vi "Call_SubPanal.vi"(8 "错误输入（无错误）":errorcluster, 10 "VI引用句柄":refnum<vi>, 11 "SubPnl引用句柄":refnum<vi>) -> (0 "错误输出":errorcluster)   [LabVIEW 2020]
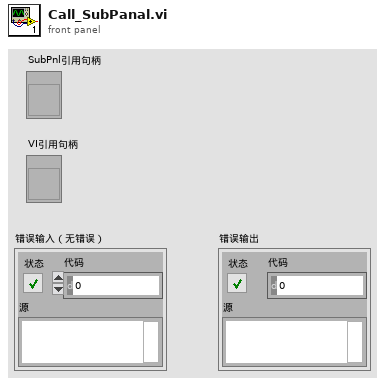
[diagram p1: front panel]
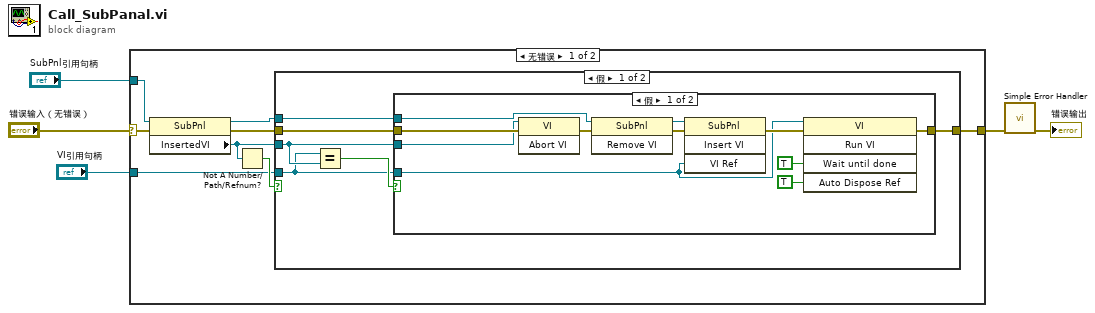
[diagram p0: block diagram]
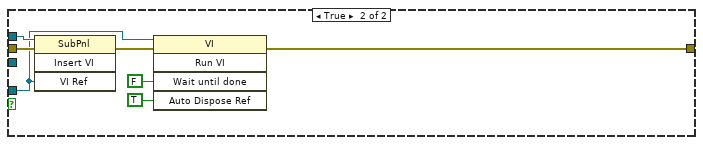
[diagram p3: hidden frame]
diagram:
  n1 = case shown="无错误" "错误输入（无错误）" {
    selector: "错误输入（无错误）" -> [w8 w39]
    tunnel: "SubPnl引用句柄" -> [w9 _]
    tunnel: "VI引用句柄" -> [w7 _]
    tunnel: [w6 w39] -> w2
    frame No Error {
      n2 = property class="SubPnl"(reference=w9, error in=w8) -> (reference out=w11:refnum<vi>, error out=w10:errorcluster, "InsertedVI"=w12:refnum<vi>)
      n3 = Not A Number/Path/Refnum?(number/path/refnum=w12) -> (NaN/Path/Refnum?=w13:bool)
      n4 = case shown="假" w13 {
        tunnel: w12 -> [w17 _]
        tunnel: w11 -> [w19 w37]
        tunnel: w10 -> [w18 w38]
        tunnel: w7 -> [w15 w35]
        tunnel: [w14 w32] -> w6
        frame False {
          n5 = Equal?(x=w15, y=w17) -> (x = y?=w16:bool)
          n6 = case shown="假" w16 {
            tunnel: w19 -> [w30 _]
            tunnel: w18 -> [w28 w31]
            tunnel: w17 -> [w27 _]
            tunnel: w15 -> [w23 _]
            tunnel: [w20 w31] -> w14
            frame False {
              n7 = invoke class="VI" method="Abort VI"(reference=w27, error in=w28) -> (error out=w29:errorcluster)  [unwired: 1 in, 2 out]
              n8 = invoke class="SubPnl" method="Remove VI"(reference=w30, error in=w29) -> (reference out=w25:refnum<vi>, error out=w26:errorcluster)  [unwired: 1 in, 1 out]
              n9 = invoke class="SubPnl" method="Insert VI"(reference=w25, error in=w26, "VI Ref"=w23) -> (error out=w24:errorcluster)  [unwired: 1 in, 3 out]
              n10 = invoke class="VI" method="Run VI"(reference=w23, error in=w24, "Wait until done"=TRUE ("结束前等待"), "Auto Dispose Ref"=TRUE ("自动销毁引用")) -> (error out=w20:errorcluster)  [unwired: 1 in, 4 out]
            }
            frame True {
            }
          }
        }
        frame True {
          n11 = invoke class="SubPnl" method="Insert VI"(reference=w37, error in=w38, "VI Ref"=w35) -> (error out=w36:errorcluster)  [unwired: 1 in, 3 out]
          n12 = invoke class="VI" method="Run VI"(reference=w35, error in=w36, "Wait until done"=FALSE ("结束前等待"), "Auto Dispose Ref"=TRUE ("自动销毁引用")) -> (error out=w32:errorcluster)  [unwired: 1 in, 4 out]
        }
      }
    }
    frame Error {
    }
  }
  n13 = call <vilib>:"Simple Error Handler.vi"("error in (no error)"=w2) -> ("error out"=→"错误输出":errorcluster)  [unwired: 4 in, 4 out]
